vi "PWM_Set_Enabled.vi"(8 "error in":errorcluster, 9 "Enable":bool=TRUE, 10 "PWM_in":T1=1 items=["Invalid"=0, "PWM1"=1, "PWM2"=2, "PWM9"=9, "PWM10"=10]) -> (0 "error out":errorcluster, 2 "PWM_out":T1 items=["Invalid"=0, "PWM1"=1, "PWM2"=2, "PWM9"=9, "PWM10"=10])   [LabVIEW 2009, in "PWM.lvlib"]
doc: "The PWM Set Enabled function block is used to enable or disable sending a continuous PWM signal to some specified PWM port. By default the function will enable it. By inputing a False value the function will disable the PWM for the selected port."
uses:
  PWM.lvlib
  PWM_Name.ctl
  <vilib>/rvi/interface/nirviReadWriteControl/nirviReadWriteControl.xnode
  FPGA Bitfiles/scmproject.lvproj_FPGA Target_RobotFPGA.vi.lvbitx
  RobotFPGA.vi
  <vilib>/Utility/error.llb/Error Cluster From Error Code.vi
  <vilib>/rvi/errors/niLvFpgaAdjustHostInterfaceError.vi
  <vilib>/rvi/interface/common/niFpgaNodeNameForErrorReporting.ctl
  <vilib>/rvi/errors/niLvFpgaWhatHappensToTopLevelVI.ctl
  niriosrv.dll
  FPGA.lvlib
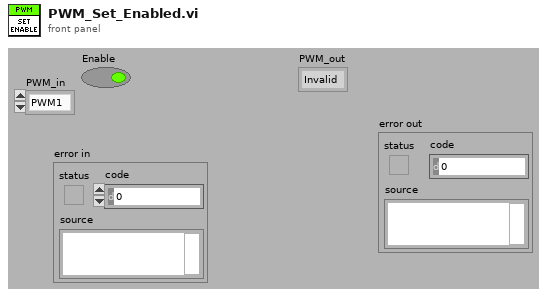
[diagram p1: front panel]
types:
  T1 = typedef "PWM.lvlib/PWM_Name.ctl" = u16
  T2 = typedef "niFpgaNodeNameForErrorReporting.ctl" = enum16{"Open FPGA VI Reference", "Read/Write Control", "Invoke Method: Abort", "Invoke Method: Acknowledge IRQ", "Invoke Method: Download", "Invoke Method: FIFO.Configure", "Invoke Method: FIFO.Read", "Invoke Method: FIFO.Start", "Invoke Method: FIFO.Stop", "Invoke Method: FIFO.Write", "Invoke Method: Reset", "Invoke Method: Run", "Invoke Method: Wait on IRQ", "Close FPGA VI Reference"}
  T3 = typedef "niLvFpgaWhatHappensToTopLevelVI.ctl" = enum16{"top level VI scripted behind XNode", "top level VI inlined behind XNode"}
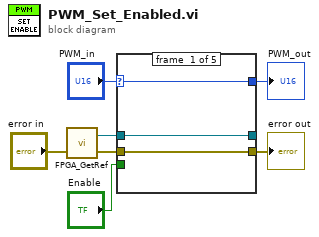
[diagram p0: block diagram]
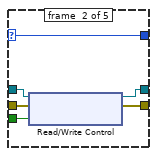
[diagram p2: hidden frame]
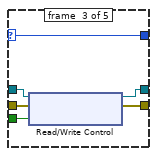
[diagram p3: hidden frame]
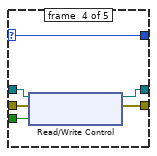
[diagram p4: hidden frame]
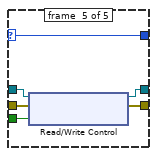
[diagram p5: hidden frame]
diagram:
  n1 = call "FPGA_GetRef.vi"("error in (no error)"="error in") -> ("error out"=w1:errorcluster, "FPGA_Ref"=w3:refnum<k20>)  [unwired: 1 in]
  n2 = case shown="0, Default" "PWM_in" {
    selector: "PWM_in" -> [w8 w11 w54 w97 w140]
    tunnel: w3 -> [w10 w14 w57 w100 w143]
    tunnel: w1 -> [w9 w16 w59 w102 w145]
    tunnel: [w10 w13 w56 w99 w142] -> _
    tunnel: [w9 w15 w58 w101 w144] -> w6
    tunnel: "Enable" -> [_ w12 w55 w98 w141]
    tunnel: [w8 w11 w54 w97 w140] -> w4
    frame #0 {
    }
    frame #1 {
      n3 = xnode "Read/Write Control"("FPGA VI Reference In"=w14, "error in"=w16, "PWM1_Enable"=w12) -> ("FPGA VI Reference Out"=w13:refnum<k20>, "error out"=w15:errorcluster)
    }
    frame #2 {
      n4 = xnode "Read/Write Control"("FPGA VI Reference In"=w57, "error in"=w59, "PWM2_Enable"=w55) -> ("FPGA VI Reference Out"=w56:refnum<k20>, "error out"=w58:errorcluster)
    }
    frame #3 {
      n5 = xnode "Read/Write Control"("FPGA VI Reference In"=w100, "error in"=w102, "PWM9_Enable"=w98) -> ("FPGA VI Reference Out"=w99:refnum<k20>, "error out"=w101:errorcluster)
    }
    frame #4 {
      n6 = xnode "Read/Write Control"("FPGA VI Reference In"=w143, "error in"=w145, "PWM10_Enable"=w141) -> ("FPGA VI Reference Out"=w142:refnum<k20>, "error out"=w144:errorcluster)
    }
  }
  "error out" <- w6
  "PWM_out" <- w4
